vi "读取数据文件.vi"(8 "错误输入":errorcluster, 11 "文件地址输入":path) -> (0 "错误输出":errorcluster, 2 "Return String":string, 3 "树莓派文件地址":string)   [LabVIEW 2019]
uses:
  SFTP Library/LabSFTP.lvlib
panel:
  out "连接的字符串":string
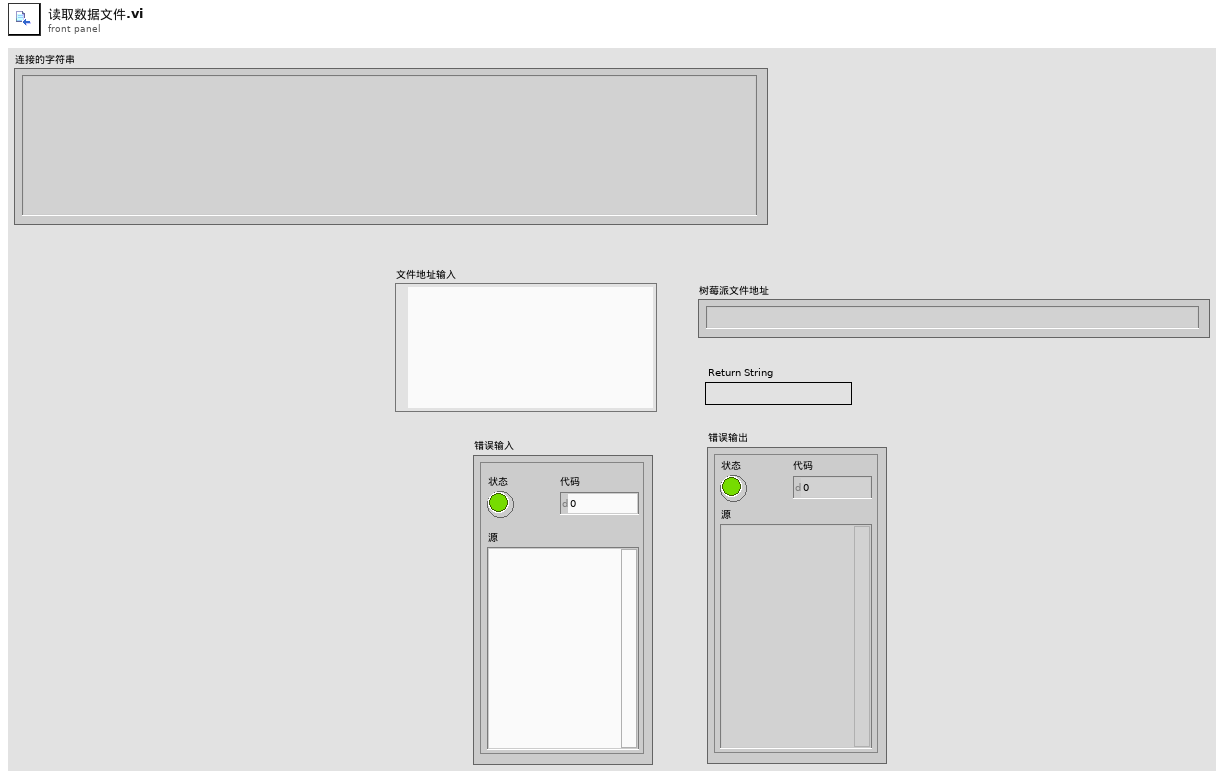
[diagram p1: front panel]
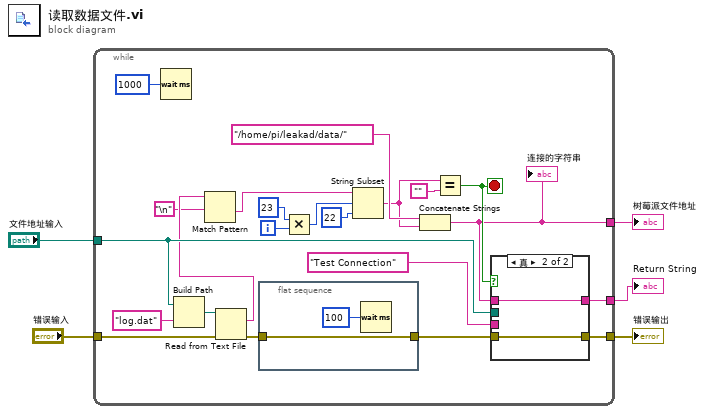
[diagram p0: block diagram]
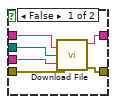
[diagram p2: hidden frame]
diagram:
  n1 = while {
    tunnel: "错误输入" -> [w16]
    tunnel: "文件地址输入" -> [w15]
    tunnel: [w10] -> w3
    tunnel: [w14] -> w2
    tunnel: [w13] -> w1
    i -> [w9]
    stop <- w12 stop-if-true
    n2 = Wait (ms)(milliseconds to wait=u32 1000 ("毫秒计时值")) -> ()  [unwired: 1 out]
    n3 = Build Path(base path=w15, name or relative path="log.dat" ("名称或相对路径")) -> (appended path=w26:path)
    n4 = Read from Text File(file (use dialog)=w26, error in=w16) -> (text=w8:string, error out=w24:errorcluster)  [unwired: 2 in, 2 out]
    n5 = Match Pattern(string=w8, regular expression="\n") -> (after substring=w6:string)  [unwired: 1 in, 3 out]
    n6 = flat-sequence {
      tunnel: w24 -> [w37]
      tunnel: [w37] -> w22
      frame #0 {
        n7 = Wait (ms)(milliseconds to wait=u32 100 ("等待时间（毫秒）")) -> ()  [unwired: 1 out]
      }
    }
    n8 = Multiply(x=23, y=w9) -> (x*y=w11:i32)
    n9 = String Subset(string=w6, offset (0)=w11, length (rest)=22 ("长度（剩余）")) -> (substring=w18:string)
    n10 = Concatenate Strings("/home/pi/leakad/data/" ("字符串"), w18) -> (w10:string)
    "连接的字符串" <- w10
    n11 = Equal?(x=w18, y="") -> (x = y?=w12:bool)
    n12 = case shown="真" w12 {
      tunnel: w22 -> [w31 w35]
      tunnel: "Test Connection" ("Connection Name") -> [w30 _]
      tunnel: w15 -> [w29 _]
      tunnel: w10 -> [w28 w34]
      tunnel: [w33 w35] -> w14
      tunnel: [w32 w34] -> w13
      frame False {
        n13 = call "Download File.vi"("error in (no error)"=w31, "Connection Name"=w30, "Local File Path"=w29, "Remote File Path"=w28) -> ("error out"=w33:errorcluster, "Return String"=w32:string)  [unwired: 6 in]
      }
      frame True {
      }
    }
  }
  "错误输出" <- w2
  "树莓派文件地址" <- w3
  "Return String" <- w1
